vi "Tree_DragDrop_Event Handler_ACAF.vi"(8 "error in (no error)":errorcluster, 11 "Tree Ref Array":refnum<vi>[](array[refnum])) -> (0 "error out":errorcluster, 3 "Tree Ref Array Out":refnum<vi>[](array[refnum]))   [LabVIEW 2023]
doc: "Launch asynchronous event handler for syncing drag and drop actions for non-indented trees."
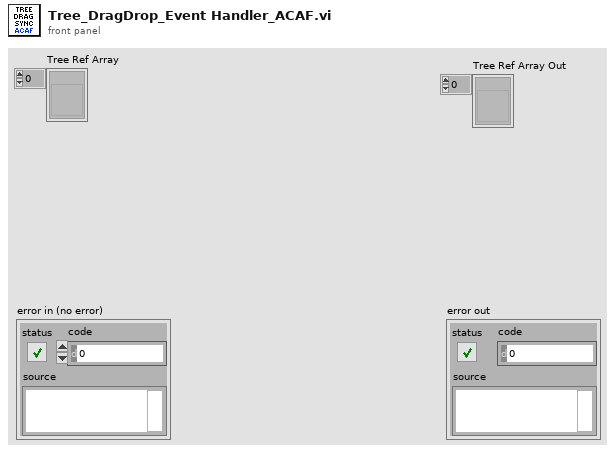
[diagram p1: front panel]
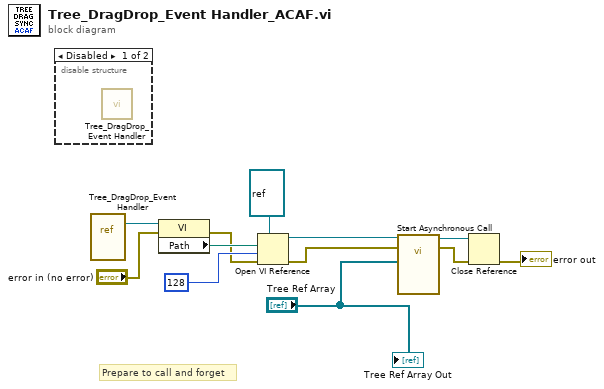
[diagram p0: block diagram]
diagram:
  # "Prepare to call and forget"
  n1 = disable-structure shown="Disabled" {
    frame Disabled {
      n2 = call "Tree_DragDrop_Event Handler.vi"() -> ()  [unwired: 12 in]
    }
    frame Enabled {
    }
  }
  n3 = vi-ref "Tree_DragDrop_Event Handler.vi"() -> (w12:refnum<vi>)
  n4 = property class="VI"(reference=w12, error in="error in (no error)") -> (error out=w1:errorcluster, "Path"=w8:path)  [unwired: 1 out]
  n5 = Open VI Reference(type specifier VI Refnum (for type only)=refnum<vi> refnum, vi path=w8, options=128, error in (no error)=w1) -> (vi reference=w3:refnum<vi>, error out=w7:errorcluster)  [unwired: 2 in]
  n6 = call-by-ref "Start Asynchronous Call"(reference=w3, error in=w7, "Tree Ref Array"="Tree Ref Array") -> (reference out=w6:refnum<vi>, error out=w5:errorcluster)  [unwired: 11 in]
  n7 = Close Reference(reference=w6, error in (no error)=w5) -> (error out=→"error out":errorcluster)
  "Tree Ref Array Out" <- "Tree Ref Array"
